vi "Main.vi"(11 "Script in":refnum<class "_Rename.lvclass">) -> ()   [LabVIEW 2021, in "_Rename.lvlib" / "_Rename.lvclass"]
uses:
  _Rename.lvclass
  _Rename.lvclass/_Rename.ctl
  <vilib>/Utility/EditLVLibs/Edit LVLibs.lvlib
  <vilib>/Utility/EditLVProj/Edit LVProj.lvlib
  _Shared/_Shared.lvlib
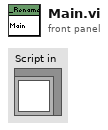
[diagram p1: front panel]
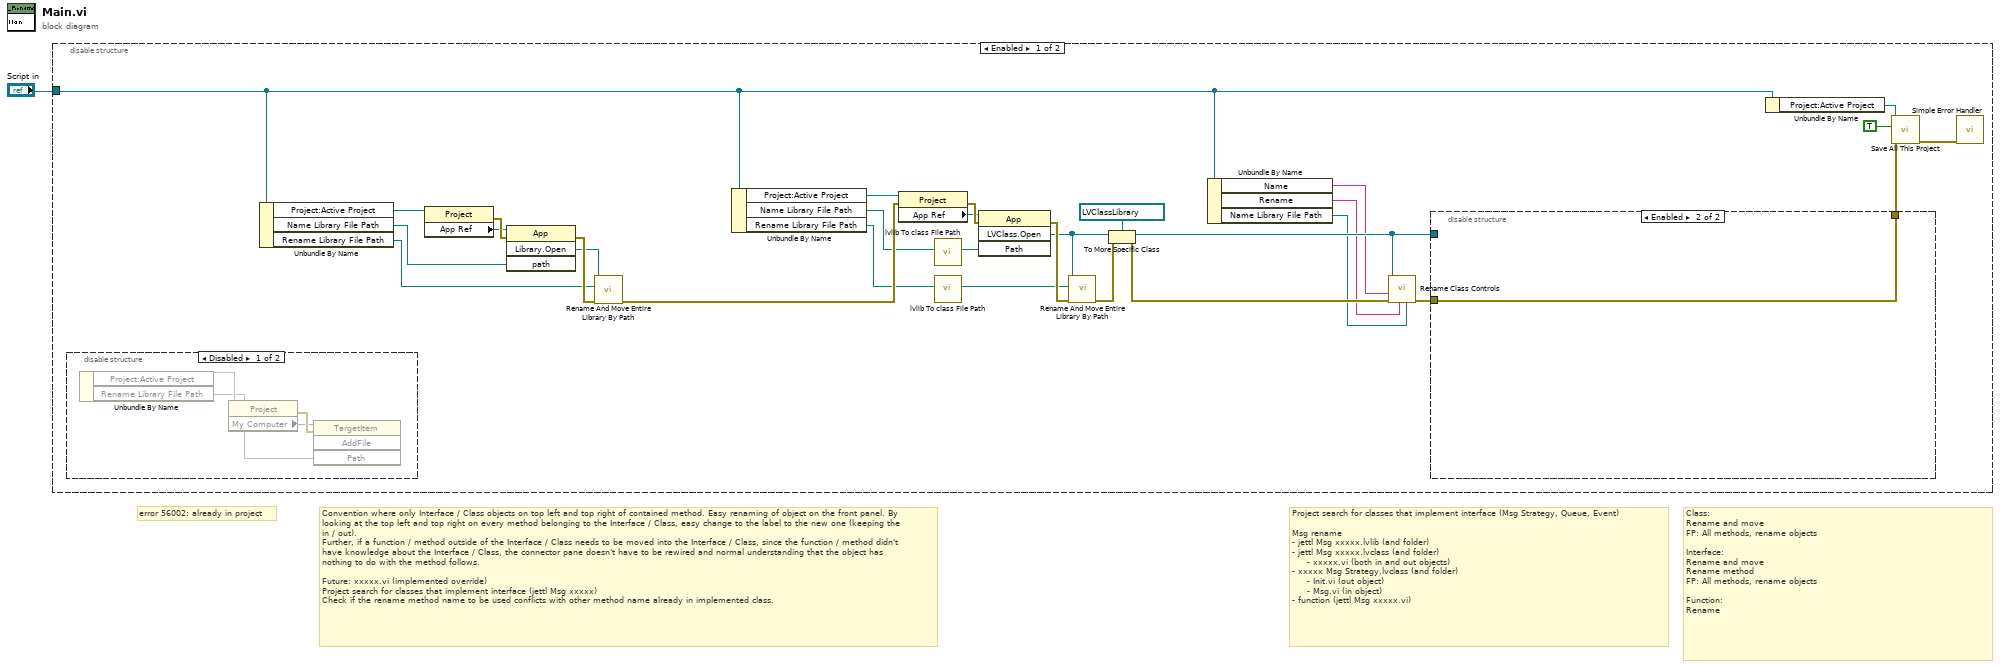
[diagram p0: block diagram]
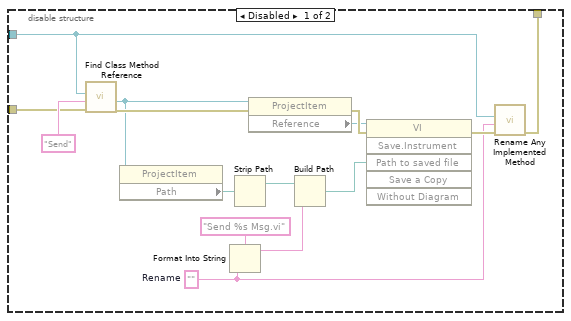
[diagram p2: hidden frame]
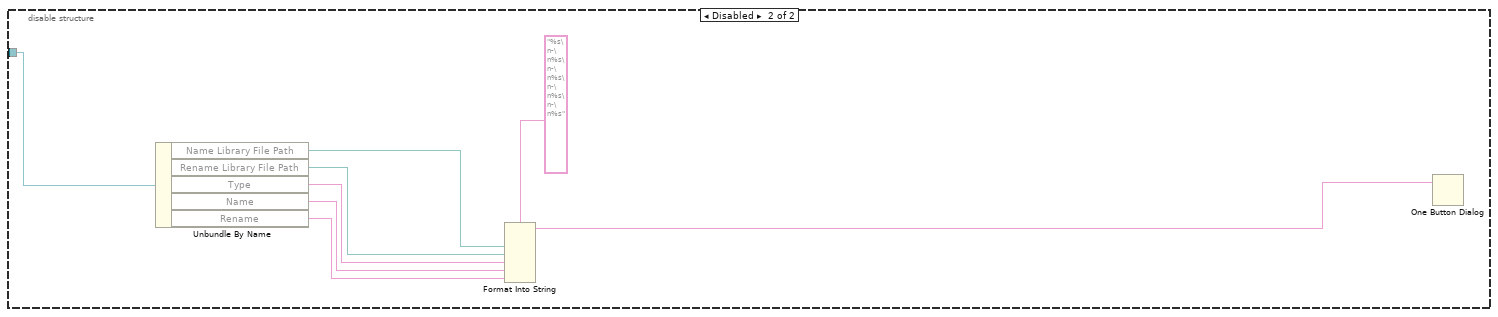
[diagram p4: hidden frame]
diagram:
  # "error 56002: already in project"
  # "Class:\nRename and move\nFP: All methods, rename objects\n\nInterface:\nRename and move\nRename method\nFP: All methods, rename objects\n\nFunction:\nRename"
  # "Convention where only Interface / Class objects on top left and top right of contained method. Easy renaming of object on the front panel. By looking at the top left and top right on every method belonging to the Interface / Class, easy change to the label to the new one (keeping the in / out).\nFurther, if a function / method outside of the Interface / Class needs to be moved into the Interface / Class, since the function / method didn't have knowledge about the Interface / Class, the connector pane doesn't have to be rewired and normal understanding that the object has nothing to do with the method follows.\n\nFuture: xxxxx.vi (implemented override)\nProject search for classes that implement interface (jettl Msg xxxxx)\nCheck if the rename method name to be used conflicts with other method name already in implemented class."
  # "Project search for classes that implement interface (Msg Strategy, Queue, Event)\n\nMsg rename\n- jettl Msg xxxxx.lvlib (and folder)\n- jettl Msg xxxxx.lvclass (and folder)\n     - xxxxx.vi (both in and out objects)\n- xxxxx Msg Strategy.lvclass (and folder)\n     - Init.vi (out object)\n     - Msg.vi (in object)\n- function (jettl Msg xxxxx.vi)"
  n1 = disable-structure shown="Enabled" {
    disable-tunnel: "Script in" -> [w2 w61]
    frame Enabled {
      n2 = disable-structure shown="Disabled" {
        frame Disabled {
          n3 = Unbundle By Name() -> (w53:refnum<class "_Rename.lvclass">, "Project:Active Project"=w49, "Rename Library File Path"=w48)
          n4 = property class="Project"(reference=w49) -> (error in=w50:errorcluster, error out=w52:errorcluster, "My Computer"=w51:refnum<vi>)  [unwired: 1 out]
          n5 = invoke class="TargetItem" method="AddFile"(reference=w51, error in=w52, "Path"=w48) -> ()  [unwired: 1 in, 4 out]
        }
        frame Enabled {
        }
      }
      n6 = Unbundle By Name(w2) -> ("Project:Active Project"=w5:refnum<vi>, "Name Library File Path"=w6:path, "Rename Library File Path"=w4:path)
      n7 = property class="Project"(reference=w5) -> (error out=w8:errorcluster, "App Ref"=w7:refnum<vi>)  [unwired: 1 in, 1 out]
      n8 = invoke class="App" method="Library.Open"(reference=w7, error in=w8, "path"=w6) -> (error out=w9:errorcluster, "Open Library"=w3:refnum<vi>)  [unwired: 1 in, 2 out]
      n9 = call <vilib>:"Rename And Move Entire Library By Path.vi"("error in (no error)"=w9, "New library path"=w4, "Library ref in"=w3) -> ("error out"=w31:errorcluster)  [unwired: 7 in, 1 out]
      n10 = Unbundle By Name(w2) -> ("Project:Active Project"=w23:refnum<vi>, "Name Library File Path"=w11:path, "Rename Library File Path"=w21:path)
      n11 = property class="Project"(reference=w23, error in=w31) -> (error out=w25:errorcluster, "App Ref"=w24:refnum<vi>)  [unwired: 1 out]
      n12 = call "lvlib To class File Path.vi"("lvlib File Path"=w11) -> ("class File Path"=w16:path)  [unwired: 10 in]
      n13 = call "lvlib To class File Path.vi"("lvlib File Path"=w21) -> ("class File Path"=w20:path)  [unwired: 10 in]
      n14 = invoke class="App" method="LVClass.Open"(reference=w24, error in=w25, "Path"=w16) -> (error out=w26:errorcluster, "LVClass.Open"=w17:refnum<vi>)  [unwired: 1 in, 2 out]
      n15 = call <vilib>:"Rename And Move Entire Library By Path.vi"("error in (no error)"=w26, "New library path"=w20, "Library ref in"=w17) -> ("error out"=w22:errorcluster)  [unwired: 7 in, 1 out]
      n16 = To More Specific Class(target class=refnum<vi> refnum ("Class in"), reference=w17, error in=w22) -> (specific class reference=w15:refnum<vi>, error out=w18:errorcluster)
      n17 = Unbundle By Name(w2) -> ("Name"=w13:string, "Rename"=w14:string, "Name Library File Path"=w12:path)
      n18 = call "Rename Class Controls.vi"("Name Library File Path"=w12, "Rename"=w14, "error in"=w18, "Name"=w13, "Rename Class Ref"=w15) -> ("error out"=w10:errorcluster)  [unwired: 6 in]
      n19 = disable-structure shown="Enabled" {
        disable-tunnel: [w46 w47] -> w28
        disable-tunnel: w10 -> [w38 w47]
        disable-tunnel: w15 -> [w32 _]
        frame Disabled {
          w33 = ""  # Rename
          n20 = call "Find Class Method Reference.vi"("error in"=w38, "Method Name"="Send" ("regular expression"), "Class To Rename"=w32) -> ("error out"=w37:errorcluster, "Method Reference"=w34:refnum<vi>)  [unwired: 7 in]
          n21 = property class="ProjectItem"(reference=w34) -> ("Path"=w40:path)  [unwired: 1 in, 2 out]
          n22 = Format Into String(format string="Send %s Msg.vi", w33) -> (resulting string=w35:string)  [unwired: 2 in, 1 out]
          n23 = Strip Path(path=w40) -> (stripped path=w44:path)  [unwired: 1 out]
          n24 = property class="ProjectItem"(reference=w34, error in=w37) -> (error out=w45:errorcluster, "Reference"=w43:refnum<vi>)  [unwired: 1 out]
          n25 = Build Path(base path=w44, name or relative path=w35) -> (appended path=w42:path)
          n26 = invoke class="VI" method="Save.Instrument"(reference=w43, error in=w45, "Path to saved file"=w42) -> (error out=w41:errorcluster)  [unwired: 3 in, 5 out]
          n27 = call "Rename Any Implemented Method.vi"("error in"=w41, "Name"=w33, "Class To Rename"=w32) -> ("error out"=w46:errorcluster)  [unwired: 8 in]
        }
        frame Enabled {
        }
      }
      n28 = Unbundle By Name(w2) -> ("Project:Active Project"=w30:refnum<vi>)
      n29 = call <vilib>:"Save All This Project.vi"("error in (no error)"=w28, "Exclude Dependencies? (F)"=TRUE, "Project in"=w30) -> ("error out"=w27:errorcluster)  [unwired: 7 in, 1 out]
      n30 = call <vilib>:"Simple Error Handler.vi"("error in (no error)"=w27) -> ()  [unwired: 4 in, 5 out]
    }
    frame Disabled {
      n31 = Unbundle By Name(w61) -> ("Name Library File Path"=w59:path, "Rename Library File Path"=w58:path, "Type"=w57:string, "Name"=w56:string, "Rename"=w55:string)
      n32 = Format Into String(format string="%s\n-\n%s\n-\n%s\n-\n%s\n-\n%s", w59, w58, w57, w56, w55) -> (resulting string=w54:string)  [unwired: 2 in, 1 out]
      n33 = One Button Dialog(message=w54) -> ()  [unwired: 1 in, 1 out]
    }
  }
